vi "jettl Msg Merge Error.vi"(10 "Error":errorcluster) -> (2 "Msg Strategy":refnum<class "Msg Strategy.lvclass">)   [LabVIEW 2021, in "jettl Msg Merge Error.lvlib"]
uses:
  jettl Msg Merge Error.lvlib
  jettl/Msg Strategy/Msg Strategy.lvclass
  Merge Error Msg Strategy/Merge Error Msg Strategy.lvclass
  C:/git/jettl/src/jettl/Msg Strategy/Msg Strategy.lvclass
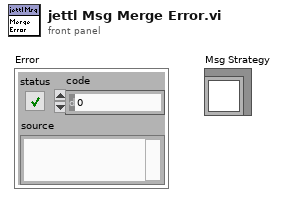
[diagram p1: front panel]
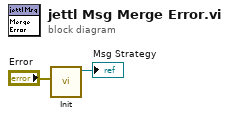
[diagram p0: block diagram]
diagram:
  n1 = call "Init.vi"("Error"="Error") -> ("Merge Error Msg Strategy out"=→"Msg Strategy":refnum<class "Merge Error Msg Strategy.lvclass">)  [unwired: 10 in]
